vi "Determine insert positions.vi"(8 "error in (no error)":errorcluster, 10 "Points to be distributed (D)":i32, 11 "Array size (N)":i32=512) -> (0 "error out":errorcluster, 3 "Distribution Indices (with one extra) - delete required end":i32[](array[numeric]))   [LabVIEW 2012]
panel:
  out "size(s)":i32
  out "Pixel Distribution (at 'zero points')":i32[](graph)
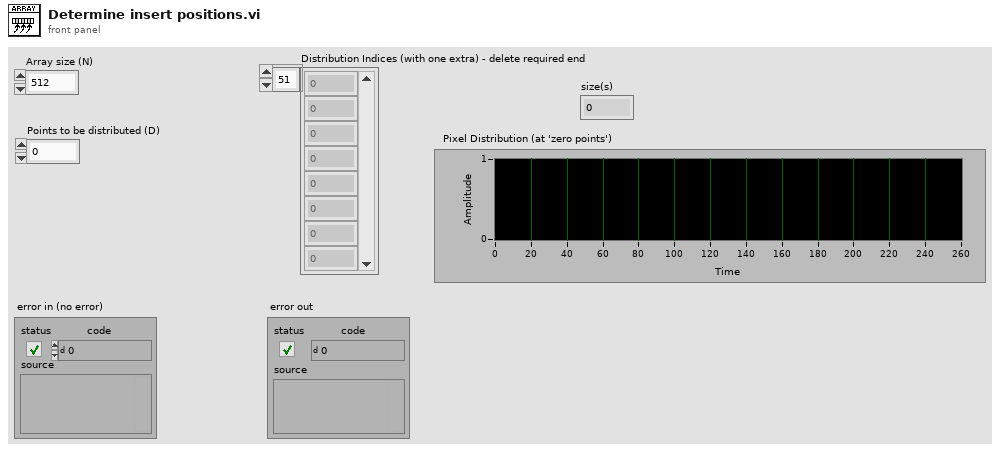
[diagram p1: front panel]
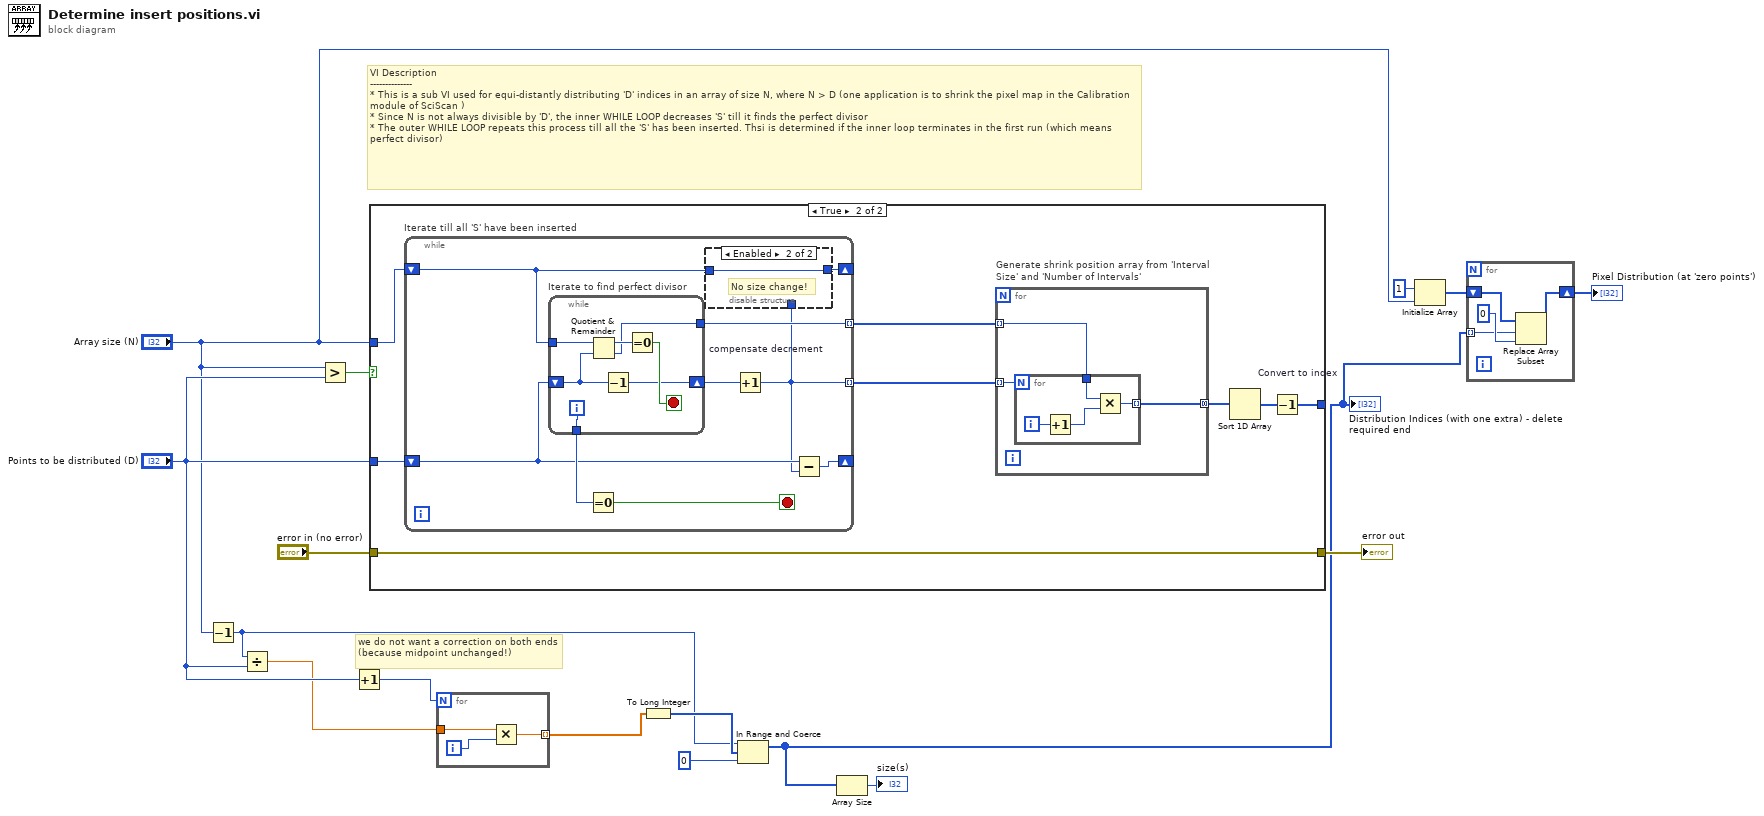
[diagram p0: block diagram]
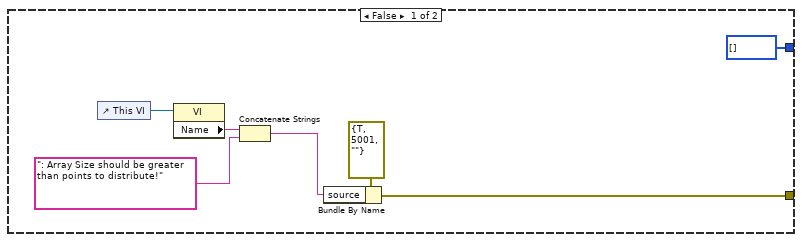
[diagram p2: hidden frame]
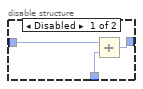
[diagram p3: hidden frame]
diagram:
  # "we do not want a correction on both ends (because midpoint unchanged!)"
  # "VI Description\n--------------\n* This is a sub VI used for equi-distantly distributing 'D' indices in an array of size N, where N > D (one application is to shrink the pixel map in the Calibration module of SciScan )\n* Since N is not always divisible by 'D', the inner WHILE LOOP decreases 'S' till it finds the perfect divisor \n* The outer WHILE LOOP repeats this process till all the 'S' has been inserted. Thsi is determined if the inner loop terminates in the first run (which means perfect divisor)"
  n1 = Decrement(x="Array size (N)") -> (x-1=w1:i32)
  n2 = Divide(x=w1, y="Points to be distributed (D)") -> (x/y=w8:dbl)
  n3 = Greater?(x="Array size (N)", y="Points to be distributed (D)") -> (0:w16:bool)
  n4 = Increment(x="Points to be distributed (D)") -> (x+1=w4:i32)
  n5 = case shown="True" w16 {
    tunnel: "Array size (N)" -> [_ w28]
    tunnel: [i32[] [] w26] -> _
    tunnel: "Points to be distributed (D)" -> [_ w25]
    tunnel: [w17 w24] -> w15
    tunnel: "error in (no error)" -> [_ w24]
    frame False {
      n6 = control-ref of="This VI"() -> (w22:refnum<vi>)
      n7 = property class="VI"(reference=w22) -> ("Name"=w21:string)  [unwired: 1 in, 2 out]
      n8 = Concatenate Strings(w21, ": Array Size should be greater than points to distribute!" ("string")) -> (w19:string)
      n9 = Bundle By Name(cluster=errorcluster {"status"=TRUE, "code"=5001, "source"=""} ("error constant"), "source"=w19) -> (w17:errorcluster)
    }
    frame True {
      n10 = while "Iterate till all 'S' have been inserted" {
        tunnel: [w39] -> w30 mode=indexing
        tunnel: [w44] -> w31 mode=indexing
        shift-right: [w43] -> _
        shift-left: w25 -> [w42]
        shift-right: [w41] -> _
        shift-left: w28 -> [w40]
        stop <- w47 stop-if-true
        n11 = while "Iterate to find perfect divisor" {
          tunnel: w40 -> [w58]
          shift-right: [w54] -> w46
          shift-left: w42 -> [w55]
          tunnel: [w53] -> w45
          tunnel: [w52] -> w44
          i -> [w53]
          stop <- w56 stop-if-true
          n12 = Quotient & Remainder(x=w58, y=w55) -> (x-y*floor(x/y)=w57:i32, floor(x/y)=w52:i32)
          n13 = Decrement(x=w55) -> (x-1=w54:i32)
          n14 = Equal To 0?(x=w57) -> (x = 0?=w56:bool)
        }
        n15 = Equal To 0?(x=w45) -> (x = 0?=w47:bool)
        n16 = Increment "compensate decrement"(x=w46) -> (x+1=w39:i32)
        n17 = disable-structure shown="Enabled" {
          disable-tunnel: [w50 w51] -> w41
          disable-tunnel: w40 -> [w49 w51]
          disable-tunnel: w39 -> [w48 _]
          frame Disabled {
            n18 = Add(x=w49, y=w48) -> (x+y=w50:i32)
          }
          frame Enabled {
            # "No size change!"
          }
        }
        n19 = Subtract(x=w42, y=w39) -> (x-y=w43:i32)
      }
      n20 = for "Generate shrink position array from 'Interval Size' and 'Number of Intervals'" {
        tunnel: w31 -> [w33] mode=indexing
        tunnel: w30 -> [w34] mode=indexing
        tunnel: [w32] -> w29 mode=concatenating
        n21 = for {
          N: w34 -> [_]
          tunnel: w33 -> [w38]
          tunnel: [w36] -> w32 mode=indexing
          i -> [w37]
          n22 = Increment(x=w37) -> (x+1=w35:i32)
          n23 = Multiply(x=w38, y=w35) -> (x*y=w36:i32)
        }
      }
      n24 = Sort 1D Array(array=w29) -> (sorted array=w27:i32[])
      n25 = Decrement "Convert to index"(x=w27) -> (x-1=w26:i32[])
    }
  }
  "error out" <- w15
  n26 = for {
    N: w4 -> [_]
    tunnel: w8 -> [w61]
    tunnel: [w59] -> w9 mode=indexing
    i -> [w60]
    n27 = Multiply(x=w61, y=w60) -> (x*y=w59:dbl)
  }
  n28 = To Long Integer(number=w9) -> (32bit integer=w5:i32[])
  n29 = In Range and Coerce(upper limit=w1, x=w5, lower limit=0) -> (coerced(x)=w3:i32[])  [unwired: 1 out]
  "Distribution Indices (with one extra) - delete required end" <- w3
  n30 = Array Size(array=w3) -> (size(s)=→"size(s)":i32)
  n31 = Initialize Array(1 ("element"), "Array size (N)") -> (w12:i32[])
  n32 = for {
    tunnel: w3 -> [w64] mode=indexing
    shift-right: [w62] -> w11
    shift-left: w12 -> [w63]
    n33 = Replace Array Subset(array=w63, new element=0 ("new element/subarray"), index=w64) -> (w62:i32[])
  }
  "Pixel Distribution (at 'zero points')" <- w11
